vi "Continuous Sweep Waveform.vi"(8 "error in (no error)":errorcluster, 9 "Sweep Index":i32, 10 "Waveforms in":waveform(dbl)[](array[waveform]), 11 "Generator in":refnum<class "Generator.lvclass">) -> (0 "error out":errorcluster, 1 "finished?":bool, 2 "Waveforms out":waveform(dbl)[](array[waveform]), 3 "Generator in":refnum<class "Generator.lvclass">)   [LabVIEW 2019, in "Generator.lvclass"]
uses:
  Generator.lvclass
  Generator.lvclass/Generator.ctl
  typedefs/Sweep.Pattern--Enum.ctl
  <vilib>/ErrorRing/Error Ring.xnode
  <vilib>/Analysis/NI_AALBase.lvlib
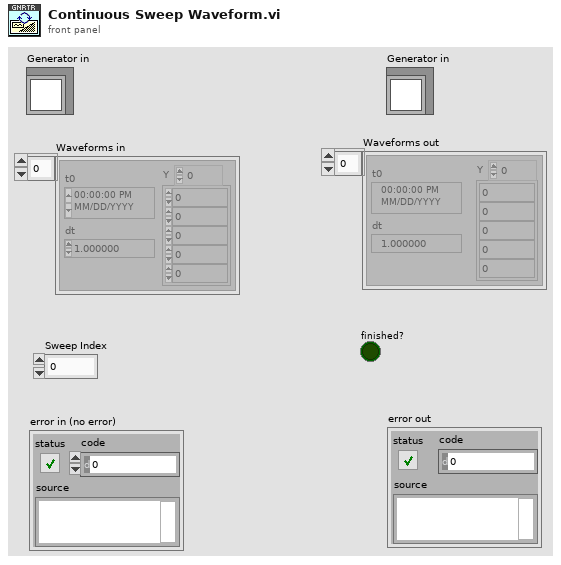
[diagram p1: front panel]
types:
  T1 = typedef "Generator.lvclass/Sweep.Pattern--Enum.ctl" = enum16{"Ramp /", "Ramp /\\", "Smooth Ramp _/", "Smooth Ramp _/\\_", "Table"}
  T2 = typedef "Generator.lvclass/AO.Channel--Cluster--Array.ctl" = T3[]
  T3 = typedef "Generator.lvclass/AO.Channel--Cluster.ctl" = cluster{"Enable?":bool, "Channel":i32, "Amplitude":dbl, "Offset":dbl, "Frequency":dbl, "Phase":dbl, "Function":T4, "Sweeping?":bool, "Limit AC?":bool, "Limit DC?":bool, "Duty Cycle?":bool, "Duty Cycle":dbl}
  T4 = typedef "Generator.lvclass/AO.Channel.Function--Enum.ctl" = enum16{"sine", "square", "triangle", "saw"}
  T5 = typedef "Generator.lvclass/Sweep.Channel--Cluster--Array.ctl" = T6[]
  T6 = typedef "Generator.lvclass/Sweep.Channel--Cluster.ctl" = cluster{"Enable?":bool, "Channel":u16, "Start":dbl, "End":dbl, "Pattern":T1, "Table":dbl[]}
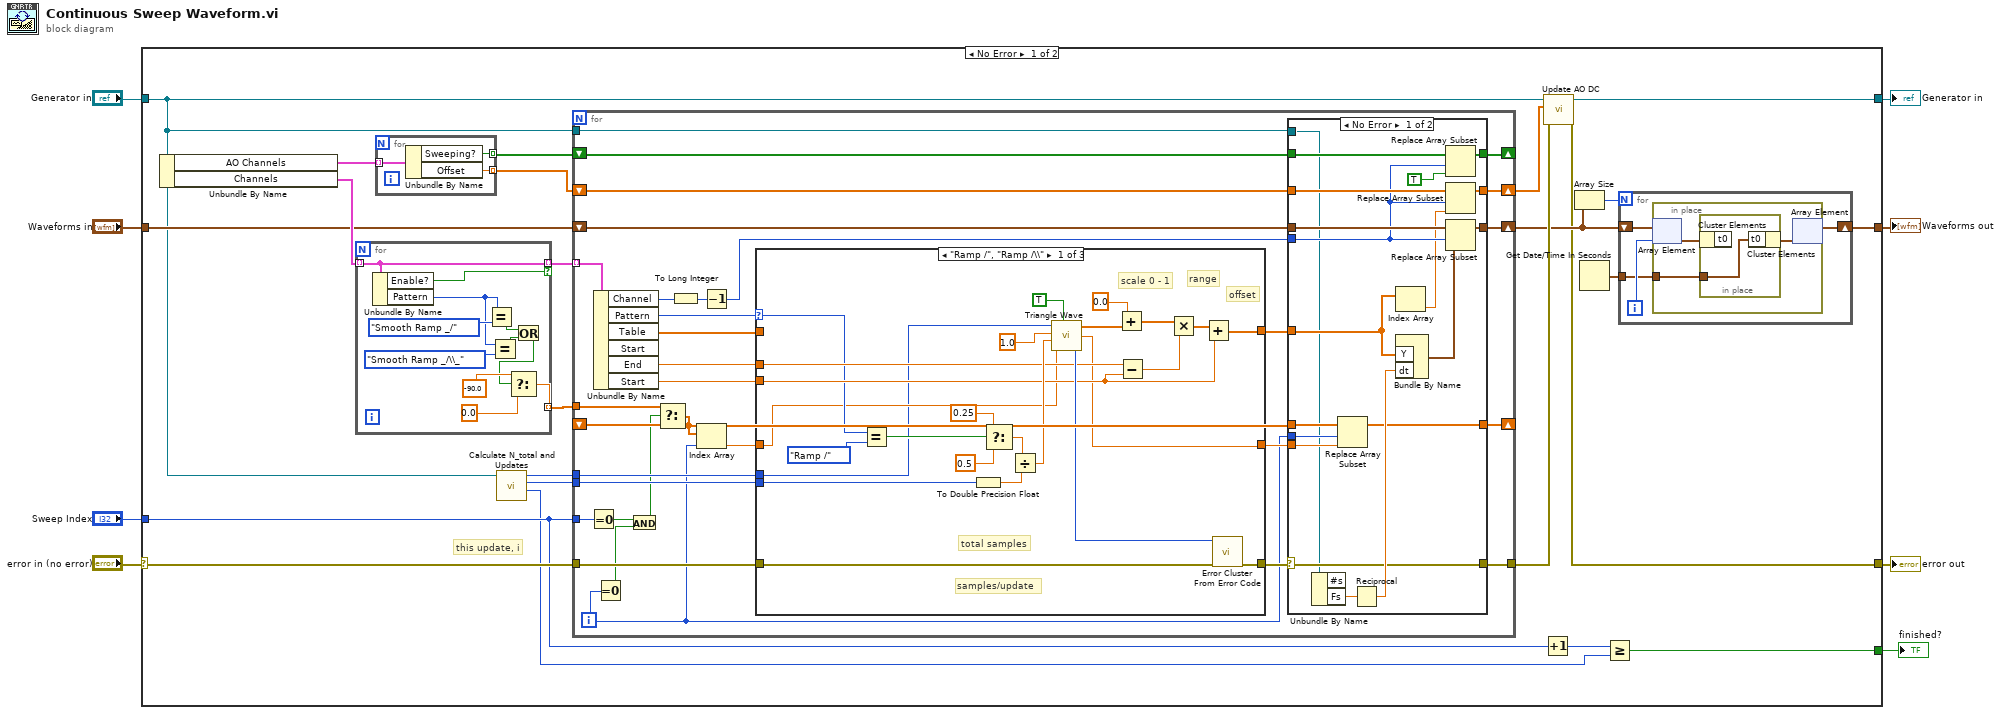
[diagram p0: block diagram]
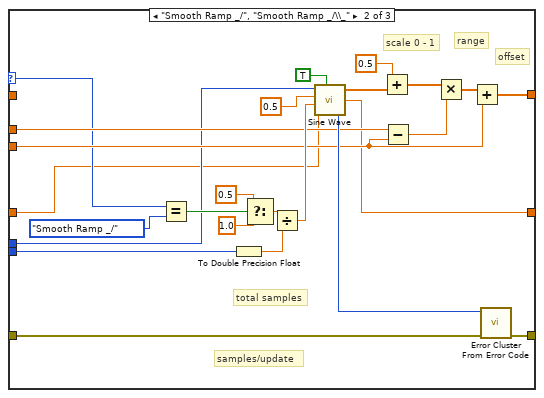
[diagram p2: hidden frame]
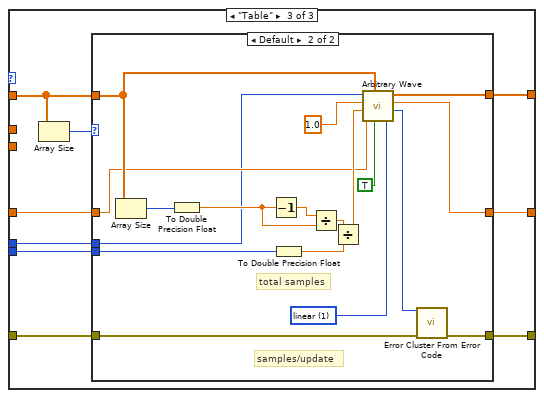
[diagram p3: hidden frame]
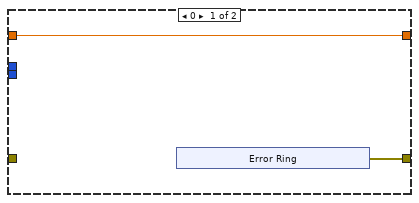
[diagram p4: hidden frame]
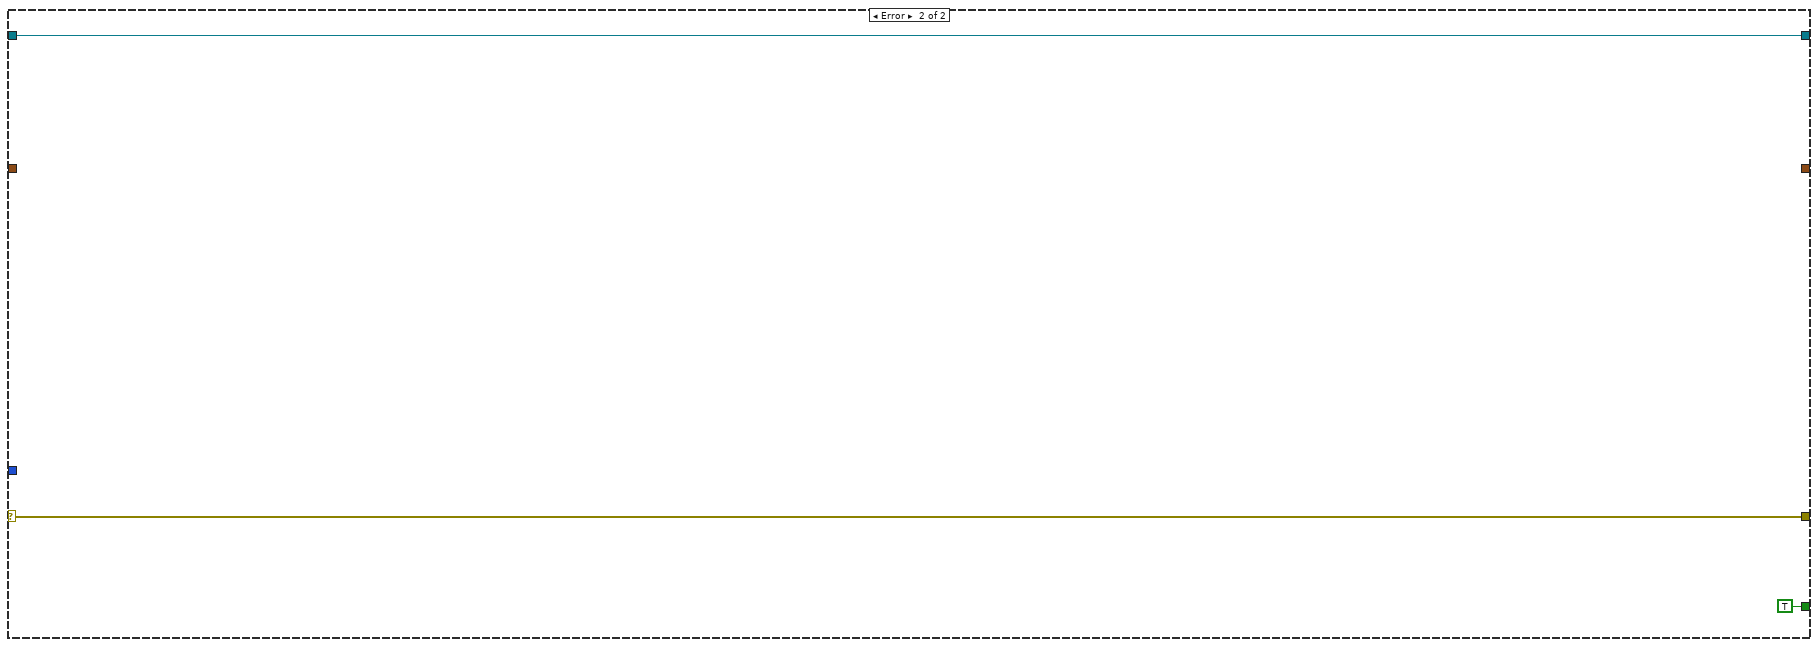
[diagram p6: hidden frame]
diagram:
  n1 = case shown="No Error" "error in (no error)" {
    selector: "error in (no error)" -> [w27 w196]
    tunnel: [w9 w196] -> w7
    tunnel: "Generator in" -> [w21 w195]
    tunnel: [w25 w195] -> w5
    tunnel: "Waveforms in" -> [w26 _]
    tunnel: [w14 _] -> w3
    tunnel: "Sweep Index" -> [w12 _]
    tunnel: [w13 TRUE] -> w1
    frame No Error {
      # "this update, i"
      n2 = Unbundle By Name(w21) -> ("AO Channels"=w28:T2, "Channels"=w31:T5)
      n3 = for {
        tunnel: w31 -> [w193] mode=indexing
        tunnel: [w193] -> w19 mode=indexing if=w192
        tunnel: [w183] -> w18 mode=indexing
        n4 = Unbundle By Name(w193) -> ("Enable?"=w192:bool, "Pattern"=w190:T1)
        n5 = Equal?(x=w190, y=Sweep.Pattern--Enum."Smooth Ramp _/" ("Pattern")) -> (x = y?=w188:bool)
        n6 = Equal?(x=w190, y=Sweep.Pattern--Enum."Smooth Ramp _/\\_" ("Pattern")) -> (x = y?=w187:bool)
        n7 = Or(x=w188, y=w187) -> (x .or. y?=w184:bool)
        n8 = Select(t=-90.0 ("phase in"), s=w184, f=0.0 ("element")) -> (s? t:f=w183:dbl)
      }
      n9 = for {
        tunnel: [w182] -> w29 mode=indexing
        tunnel: [w181] -> w30 mode=indexing
        tunnel: w28 -> [w180] mode=indexing
        n10 = Unbundle By Name(w180) -> ("Sweeping?"=w181:bool, "Offset"=w182:dbl)
      }
      n11 = call "Calculate N_total and Updates.vi"("Generator in"=w21) -> ("Updates"=w10:i32, "Total Samples"=w20:i32, "Samples/Update"=w22:i32)  [unwired: 8 in]
      n12 = for {
        tunnel: w19 -> [w56] mode=indexing
        shift-right: [w67] -> _
        shift-left: w30 -> [w66]
        shift-right: [w64] -> w23
        shift-left: w29 -> [w65]
        shift-right: [w62] -> w15
        shift-left: w26 -> [w63]
        tunnel: w27 -> [w71]
        tunnel: [w55] -> w24
        tunnel: w12 -> [w50]
        shift-right: [w52] -> _
        shift-left: _ -> [w47]
        tunnel: w18 -> [w49]
        tunnel: w22 -> [w46]
        tunnel: w21 -> [w45]
        tunnel: w20 -> [w44]
        i -> [w43]
        n13 = Equal To 0?(x=w50) -> (x = 0?=w42:bool)
        n14 = Unbundle By Name(w56) -> ("Channel"=w60:u16, "Pattern"=w69:T1, "Table"=w70:dbl[], "End"=w68:dbl, "Start"=w58:dbl)  [unwired: 1 out]
        n15 = Equal To 0?(x=w43) -> (x = 0?=w41:bool)
        n16 = And(x=w42, y=w41) -> (x .and. y?=w40:bool)
        n17 = Select(t=w49, s=w40, f=w47) -> (s? t:f=w48:dbl[])
        n18 = To Long Integer(number=w60) -> (32bit integer=w61:i32)
        n19 = Index Array(array=w48, index=w43) -> (element=w51:dbl)
        n20 = Decrement(x=w61) -> (x-1=w59:i32)
        n21 = case shown="\"Ramp /\", \"Ramp /\\\\\"" w69 {
          selector: w69 -> [w77 w103 _]
          tunnel: w68 -> [w85 w110 _]
          tunnel: [w88 w113 w128] -> w57
          tunnel: [w95 w120 w129] -> w54
          tunnel: w71 -> [w96 w121 w130]
          tunnel: w70 -> [_ _ w126]
          tunnel: w58 -> [w83 w108 _]
          tunnel: [w75 w102 w125] -> w53
          tunnel: w51 -> [w76 w98 w124]
          tunnel: w46 -> [w74 w100 w123]
          tunnel: w44 -> [w73 w99 w122]
          frame "Ramp /", "Ramp /\\" {
            # "range"
            # "total samples"
            # "samples/update"
            # "offset"
            # "scale 0 - 1"
            n22 = Equal?(x=w77, y=Sweep.Pattern--Enum."Ramp /" ("Pattern")) -> (x = y?=w79:bool)
            n23 = To Double Precision Float(number=w73) -> (double precision float=w86:dbl)
            n24 = Select(t=0.25, s=w79, f=0.5) -> (s? t:f=w80:dbl)
            n25 = Divide(x=w80, y=w86) -> (x/y=w87:dbl)
            n26 = call <vilib>:"Triangle Wave.vi"("samples"=w74, "amplitude"=1.0, "frequency"=w87, "phase in"=w76, "reset phase"=TRUE) -> ("triangle wave"=w89:dbl[], "phase out"=w75:dbl, "error"=w90:i32)
            n27 = Add(x=0.0 ("cycles 2"), y=w89) -> (x+y=w93:dbl[])
            n28 = Subtract(x=w85, y=w83) -> (x-y=w84:dbl)
            n29 = Multiply(x=w93, y=w84) -> (x*y=w92:dbl[])
            n30 = Add(x=w92, y=w83) -> (x+y=w88:dbl[])
            n31 = call <vilib>:"Error Cluster From Error Code.vi"("error in (no error)"=w96, "error code (0)"=w90) -> ("error out"=w95:errorcluster)  [unwired: 7 in]
          }
          frame "Smooth Ramp _/", "Smooth Ramp _/\\_" {
            # "range"
            # "total samples"
            # "samples/update"
            # "offset"
            # "scale 0 - 1"
            n32 = Equal?(x=w103, y=Sweep.Pattern--Enum."Smooth Ramp _/" ("Pattern")) -> (x = y?=w104:bool)
            n33 = To Double Precision Float(number=w99) -> (double precision float=w111:dbl)
            n34 = Select(t=0.5, s=w104, f=1.0) -> (s? t:f=w105:dbl)
            n35 = Divide(x=w105, y=w111) -> (x/y=w112:dbl)
            n36 = call <vilib>:"Sine Wave.vi"("samples"=w100, "amplitude"=0.5, "frequency"=w112, "phase in"=w98, "reset phase"=TRUE) -> ("sine wave"=w114:dbl[], "phase out"=w102:dbl, "error"=w115:i32)
            n37 = Add(x=0.5 ("cycles 2"), y=w114) -> (x+y=w118:dbl[])
            n38 = Subtract(x=w110, y=w108) -> (x-y=w109:dbl)
            n39 = Multiply(x=w118, y=w109) -> (x*y=w117:dbl[])
            n40 = Add(x=w117, y=w108) -> (x+y=w113:dbl[])
            n41 = call <vilib>:"Error Cluster From Error Code.vi"("error in (no error)"=w121, "error code (0)"=w115) -> ("error out"=w120:errorcluster)  [unwired: 7 in]
          }
          frame "Table" {
            n42 = Array Size(array=w126) -> (size(s)=w127:i32)
            n43 = case shown="Default" w127 {
              tunnel: w130 -> [_ w155]
              tunnel: [w132 w154] -> w129
              tunnel: w126 -> [_ w149]
              tunnel: [_ w151] -> w128
              tunnel: [w131 w142] -> w125
              tunnel: w124 -> [w131 w141]
              tunnel: w123 -> [_ w140]
              tunnel: w122 -> [_ w139]
              frame 0 {
                n44 = xnode "Error Ring"() -> ("error out"=w132:errorcluster)
              }
              frame Default {
                w150 = 1 items=["none", "linear"] ("interpolation")
                # "total samples"
                # "samples/update"
                n45 = Array Size(array=w149) -> (size(s)=w148:i32)
                n46 = To Double Precision Float(number=w148) -> (double precision float=w143:dbl)
                n47 = Decrement(x=w143) -> (x-1=w144:dbl)
                n48 = To Double Precision Float(number=w139) -> (double precision float=w147:dbl)
                n49 = Divide(x=w144, y=w143) -> (x/y=w146:dbl)
                n50 = Divide(x=w146, y=w147) -> (x/y=w145:dbl)
                n51 = call <vilib>:"Arbitrary Wave.vi"("interpolation"=w150, "reset phase"=TRUE, "Wave Table"=w149, "phase in"=w141, "frequency"=w145, "amplitude"=1.0, "samples"=w140) -> ("error"=w152:i32, "phase out"=w142:dbl, "arbitrary wave"=w151:dbl[])
                n52 = call <vilib>:"Error Cluster From Error Code.vi"("error in (no error)"=w155, "error code (0)"=w152) -> ("error out"=w154:errorcluster)  [unwired: 7 in]
              }
            }
          }
        }
        n53 = case shown="No Error" w54 {
          selector: w54 -> [w161 w179]
          tunnel: [w173 w176] -> w67
          tunnel: w66 -> [w172 w176]
          tunnel: w65 -> [w171 w177]
          tunnel: [w170 w177] -> w64
          tunnel: w63 -> [w169 w178]
          tunnel: [w168 w178] -> w62
          tunnel: w59 -> [w167 _]
          tunnel: w57 -> [w162 _]
          tunnel: [w161 w179] -> w55
          tunnel: w53 -> [w160 _]
          tunnel: w43 -> [w159 _]
          tunnel: w48 -> [w158 w175]
          tunnel: [w157 w175] -> w52
          tunnel: w45 -> [w156 _]
          frame No Error {
            n54 = Unbundle By Name(w156) -> ("Fs"=w164:dbl)  [unwired: 1 out]
            n55 = Replace Array Subset(array=w158, new element=w160, index=w159) -> (w157:dbl[])
            n56 = Reciprocal(x=w164) -> (1/x=w163:dbl)
            n57 = Index Array(array=w162) -> (element=w166:dbl)  [unwired: 1 in]
            n58 = Bundle By Name("Y"=w162, "dt"=w163) -> (w165:waveform(dbl))  [unwired: 1 in]
            n59 = Replace Array Subset(array=w172, new element=TRUE ("new element/subarray"), index=w167) -> (w173:bool[])
            n60 = Replace Array Subset(array=w171, new element=w166, index=w167) -> (w170:dbl[])
            n61 = Replace Array Subset(array=w169, new element=w165, index=w167) -> (w168:waveform(dbl)[])
          }
          frame Error {
          }
        }
      }
      n62 = Increment(x=w12) -> (x+1=w11:i32)
      n63 = call "Update AO DC.vi"("error in (no error)"=w24, "AO.DC (V)"=w23, "Generator in"=w21) -> ("error out"=w9:errorcluster, "Generator out"=w25:refnum<class "Generator.lvclass">)  [unwired: 7 in]
      n64 = Array Size(array=w15) -> (size(s)=w16:i32)
      n65 = Get Date/Time In Seconds() -> (seconds since 1Jan1904=w17:timestamp)
      n66 = Greater Or Equal?(x=w11, y=w10) -> (x >= y?=w13:bool)
      n67 = for {
        N: w16 -> [_]
        shift-right: [w34] -> w14
        shift-left: w15 -> [w35]
        tunnel: w17 -> [w32]
        i -> [w33]
        n68 = in-place {
          in-place-border: w32 -> [w37]
          n69 = in-place-array #1(w35, w33) -> (w38:waveform(dbl))
          n70 = in-place {
            in-place-border: w37 -> [w39]
            n71 = in-place-cluster #2(w38) -> ()  [unwired: 1 out]
            n72 = in-place-cluster #2("t0"=w39) -> (w36:waveform(dbl))
          }
          n73 = in-place-array #1(w36) -> (w34:waveform(dbl)[])  [unwired: 1 out]
        }
      }
    }
    frame Error {
    }
  }
  "error out" <- w7
  "Generator in" <- w5
  "Waveforms out" <- w3
  "finished?" <- w1
